vi "Unibot - Nonlinear Model.vi"(0 "initial theta1":dbl=3.1416, 1 "initial velocity theta1":dbl, 2 "initial velocity theta2":dbl, 3 "M1":dbl=0.463901, 4 "M2":dbl=0.364069, 5 "initial theta2":dbl, 7 "Torque (Tau)":dbl, 9 "J1":dbl=0.00894463, 11 "J2":dbl=0.00251451, 12 "friction coefficient 1":dbl=0.02, 13 "friction coefficient 2":dbl=0.00109561, 14 "Amplifier Gain":dbl=0.4) -> (6 "theta1":dbl=0.11676928692181643, 8 "theta2":dbl=-0.3578561321200968, 10 "states":dbl[](array[numeric])=[0.11676928692181643, -0.3578561321200968, -0.19175807659191071, 0.3912657493379608])   [LabVIEW 2012]
uses:
  <vilib>/Simulation/Implementation/Shared/SIMSCR Execution Mode.ctl
  <vilib>/Simulation/Scripting/Companion Diagram/SimConfigNode/SimParams.ctl
  <vilib>/Simulation/Scripting/Companion Diagram/SimConfigNode/_simSolvers.ctl
  <vilib>/Simulation/Param Hierarchy/Typedefs/SIMPH Param Control Actions.ctl
  <vilib>/Simulation/Implementation/Shared/SIM limit type.ctl
  <vilib>/Simulation/Implementation/Shared/NILVSim_ParamChanged.vi
  <vilib>/Simulation/ContinuousLinear/Implementation/NILVSim Integrator new.llb/SIM Integrator distributor (scalar).vi
  <vilib>/Simulation/ContinuousLinear/Implementation/NILVSim Integrator new.llb/SIM Integrator collector (scalar).vi
  <vilib>/Simulation/Implementation/Shared/NILVSim_Manager.vi
  <vilib>/Simulation/Implementation/Shared/NILVSim_FinalizeModel.vi
  <vilib>/Simulation/Implementation/Shared/SIM Unbundle Sim Info.vi
  <vilib>/Utility/error.llb/Clear Errors.vi
  <vilib>/Simulation/Implementation/Shared/NILVSim_GetModelError.vi
  <vilib>/Simulation/Implementation/Shared/SIM SimErrorHandler.vi
  <vilib>/Simulation/Implementation/Shared/SIM Bundle Sim Info.vi
  <vilib>/Simulation/Implementation/Shared/SIMSH Read Queue.vi
  <vilib>/Simulation/Implementation/Shared/NILVSim_Initialize.vi
  <vilib>/Simulation/Utility/Implementation/NILVSim Get Time and IsAcceptedStep.vi
  <vilib>/Simulation/Scripting/Companion Diagram/SimConfigNode/SimDog.xnode
  <vilib>/Simulation/Implementation/XNodeFramework/SimXNode/SimX.xnode
  <vilib>/Simulation/ContinuousLinear/Implementation/NILVSim Integrator new.llb/SIM Integrator (scalar).vi
  <vilib>/ptbypt/NI_PtbyPt.lvlib
  <vilib>/Simulation/Implementation/Shared/NI_SIM_Implementation.lvlib
panel:
  out "B4":dbl=0.290250432
  out "B3":dbl=0.006213312
  out "B2":dbl=0.005776684800000001
  out "B1":dbl=0.006213312
  out "A4":dbl=1.00393578
  out "A3":dbl=0.006213312
  out "A2":dbl=0.006213312
  out "A1":dbl=0.01776728
  in  "g":dbl=9.81
  in  "lG1":dbl=0.116
  in  "lG2":dbl=0.134
  in  "l1":dbl=0.21
  # "Legend: \nC.G.  - Center of Gravity\nl       - Length (m)\nJ      - Moment of Inertia (kg(m^2)\nM     - Mass (kg)"
  # "Derived Parameters"
  # "C.G.2"
  # "C.G.1"
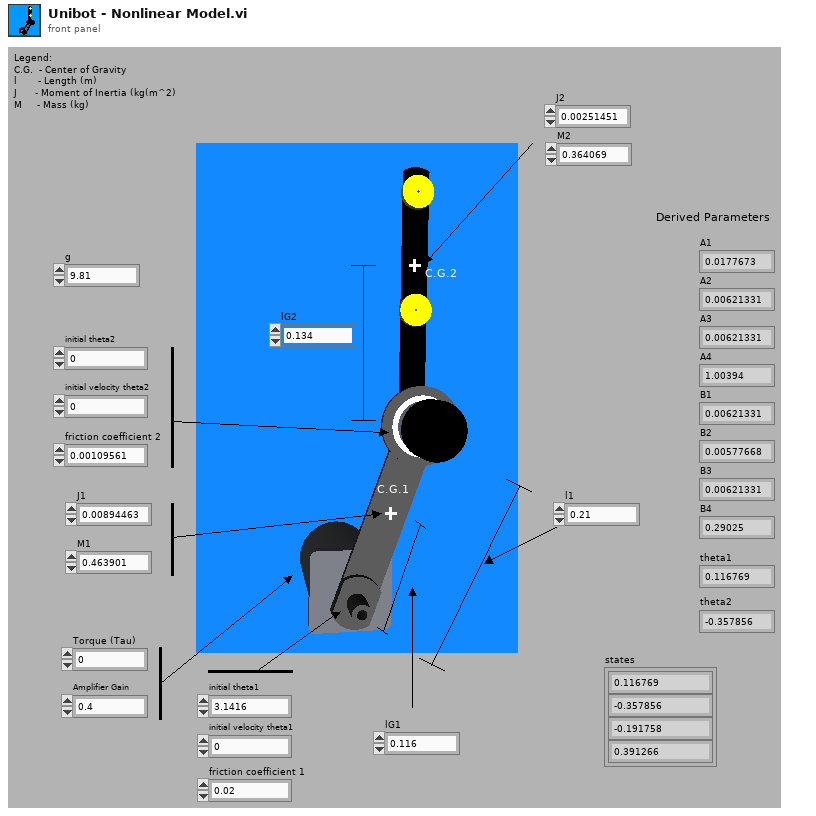
[diagram p1: front panel]
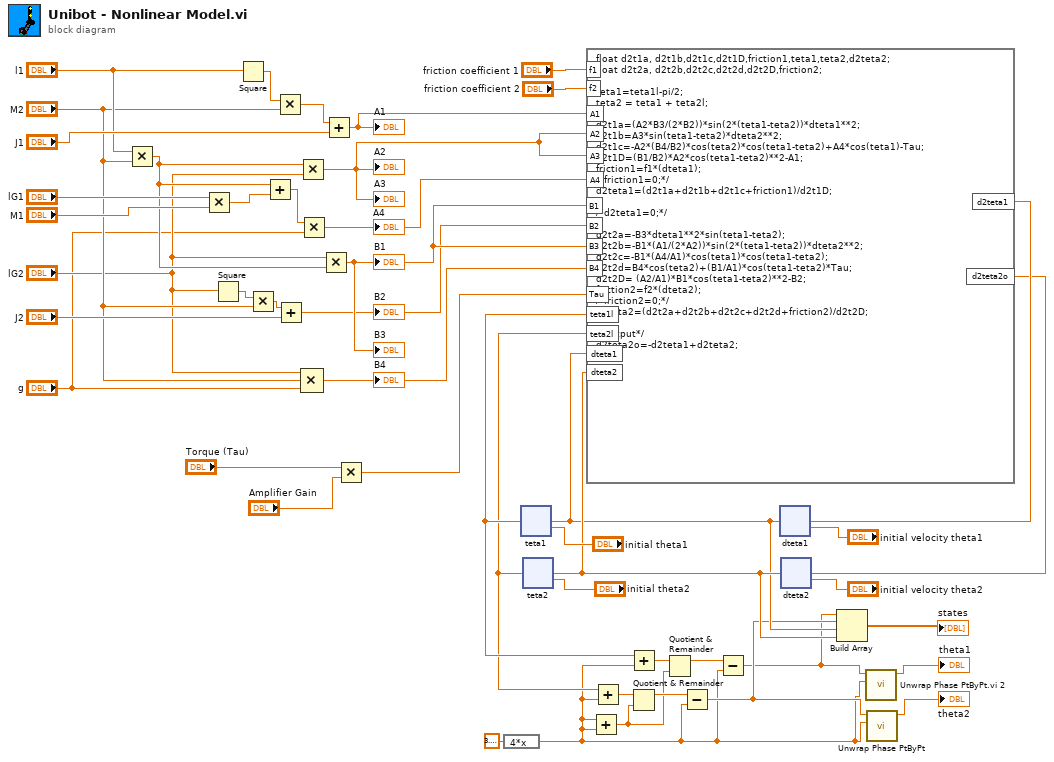
[diagram p0: block diagram]
diagram:
  n1 = Multiply ("Multiply 2")(x="l1", y="M2") -> (x*y=w37:dbl)
  n2 = Multiply ("Multiply 4")(x="lG1", y="M1") -> (x*y=w44:dbl)
  n3 = Square ("Square 2")(x="lG2") -> (x^2=w40:dbl)
  n4 = Square(x="l1") -> (x^2=w47:dbl)
  n5 = Multiply ("Multiply 7")(x=w40, y="M2") -> (x*y=w39:dbl)
  n6 = Add ("Add 2")(x=w37, y=w44) -> (x+y=w41:dbl)
  n7 = Multiply(x=w47, y="M2") -> (x*y=w46:dbl)
  n8 = Add ("Add 3")(x=w39, y="J2") -> (x+y=w23:dbl)
  "B2" <- w23
  n9 = Multiply ("Multiply 3")(x=w37, y="lG2") -> (x*y=w32:dbl)
  "A2" <- w32
  "A3" <- w32
  n10 = Multiply ("Multiply 5")(x=w41, y="g") -> (x*y=w31:dbl)
  "A4" <- w31
  n11 = Compound Arithmetic op=MULTIPLY("lG2", "M2", "g") -> (w28:dbl)
  "B4" <- w28
  n12 = Multiply ("Multiply 6")(x="lG2", y=w37) -> (x*y=w30:dbl)
  "B1" <- w30
  "B3" <- w30
  n13 = Add(x=w46, y="J1") -> (x+y=w33:dbl)
  "A1" <- w33
  n14 = Multiply ("Multiply 8")(x="Torque (Tau)", y="Amplifier Gain") -> (x*y=w22:dbl)
  n15 = expression code="4*x"(3.141592653589793 ("Constant")) -> (w1:dbl)
  n16 = Add ("Add 6")(x=w1, y=w1) -> (x+y=w6:dbl)
  n17 = xnode "teta1"("input"=w14, "initial condition"="initial theta1") -> ("output"=w9:dbl)  [unwired: 8 in, 2 out]
  n18 = Add ("Add 5")(x=w9, y=w1) -> (x+y=w10:dbl)
  n19 = Quotient & Remainder ("Quotient & Remainder 2")(x=w10, y=w6) -> (x-y*floor(x/y)=w11:dbl)  [unwired: 1 out]
  n20 = Subtract ("Subtract 2")(x=w11, y=w1) -> (x-y=w3:dbl)
  n21 = call "Unwrap Phase PtByPt.vi 2"("wrap base"=w1, "phase"=w3) -> ("unwrapped phase"=→"theta1":dbl)  [unwired: 9 in]
  n22 = xnode "teta2"("input"=w15, "initial condition"="initial theta2") -> ("output"=w8:dbl)  [unwired: 8 in, 2 out]
  n23 = Add ("Add 4")(x=w8, y=w1) -> (x+y=w13:dbl)
  n24 = Quotient & Remainder(x=w13, y=w6) -> (x-y*floor(x/y)=w12:dbl)  [unwired: 1 out]
  n25 = Subtract(x=w12, y=w1) -> (x-y=w5:dbl)
  n26 = call <vilib>:"Unwrap Phase PtByPt.vi"("wrap base"=w1, "phase"=w5) -> ("unwrapped phase"=→"theta2":dbl)  [unwired: 9 in]
  n27 = formula code="float d2t1a, d2t1b,d2t1c,d2t1D,friction1,teta1,teta2,d2teta2;\nfloat d2t2a, d2t2b,d2t2c,d2t2d,d2t2D,friction2;\n\nteta1=teta1l-pi/2;\nteta2 = teta1 + teta2l;\n\nd2t1a=(A2*B3/(2*B2))*sin(2*(teta1-teta2))*dteta1**2;\nd2t1b=A3*sin(teta1-teta2)*dteta2**2;\nd2t1c=-A2*(B4/B2)*cos(teta2)*cos(teta1-teta2)+A4*cos(teta1)-Tau;\nd2t1D=(B1/B2)*A2*cos(teta1-teta2)**2-A1;\nfriction1=f1*(dteta1);\n/*friction1=0;*/\nd2teta1=(d2t1a+d2t1b+d2t1c+friction1)/d2t1D;\n\n/*d2teta1=0;*/\n\nd2t2a=-B3*dteta1**2*sin(teta1-teta2);\nd2t2b=-B1*(A1/(2*A2))*sin(2*(teta1-teta2))*dteta2**2;\nd2t2c=-B1*(A4/A1)*cos(teta1)*cos(teta1-teta2);\nd2t2d=B4*cos(teta2)+(B1/A1)*cos(teta1-teta2)*Tau;\nd2t2D= (A2/A1)*B1*cos(teta1-teta2)**2-B2;\nfriction2=f2*(dteta2);\n/*friction2=0;*/\nd2teta2=(d2t2a+d2t2b+d2t2c+d2t2d+friction2)/d2t2D;\n\n/*output*/\nd2teta2o=-d2teta1+d2teta2;"("A1"=w33, "A2"=w32, "A3"=w32, "A4"=w31, "B1"=w30, "B2"=w23, "B3"=w30, "B4"=w28, "Tau"=w22, "teta1l"=w9, "teta2l"=w8, "dteta1"=w14, "dteta2"=w15, "f1"="friction coefficient 1", "f2"="friction coefficient 2") -> ("d2teta1"=w29:dbl, "d2teta2o"=w27:dbl)
  n28 = xnode "dteta1"("input"=w29, "initial condition"="initial velocity theta1") -> ("output"=w14:dbl)  [unwired: 8 in, 2 out]
  n29 = xnode "dteta2"("input"=w27, "initial condition"="initial velocity theta2") -> ("output"=w15:dbl)  [unwired: 8 in, 2 out]
  n30 = Build Array(w3, w5, w14, w15) -> (→"states":dbl[])
